vi "Autonomous Independent.vi"   [LabVIEW 2017]
doc: "This VI is called when autonomous begins, and will automatically be terminated when autonomous ends. You can carry out timed or sensor driven robot movement independently without needing to return to the caller."
uses:
  <vilib>/Rock Robotics/WPI/Utilities/WPI_GetSetVariantRefNum.vi
  Robot Global Data.vi
panel:
  # "Be sure to right-click and choose Data Operations>>Make Current Value default if you want to save the array values with the VI"
types:
  T1 = enum16{"Manual", "Turn For Angle", "Drive For Distance", "Motion Profile", "Recorded Auto File"}
  T2 = enum16{"Manual", "Turn For Angle", "Drive For Distance", "Motion Profile"}
  T3 = typedef "WPI_JoystickDevRef.ctl" = cluster{"Device":T4}
  T4 = typedef "WPI_JoystickDeviceEnum.ctl" = enum16{"USB 0", "USB 1", "USB 2", "USB 3", "USB 4", "USB 5"}
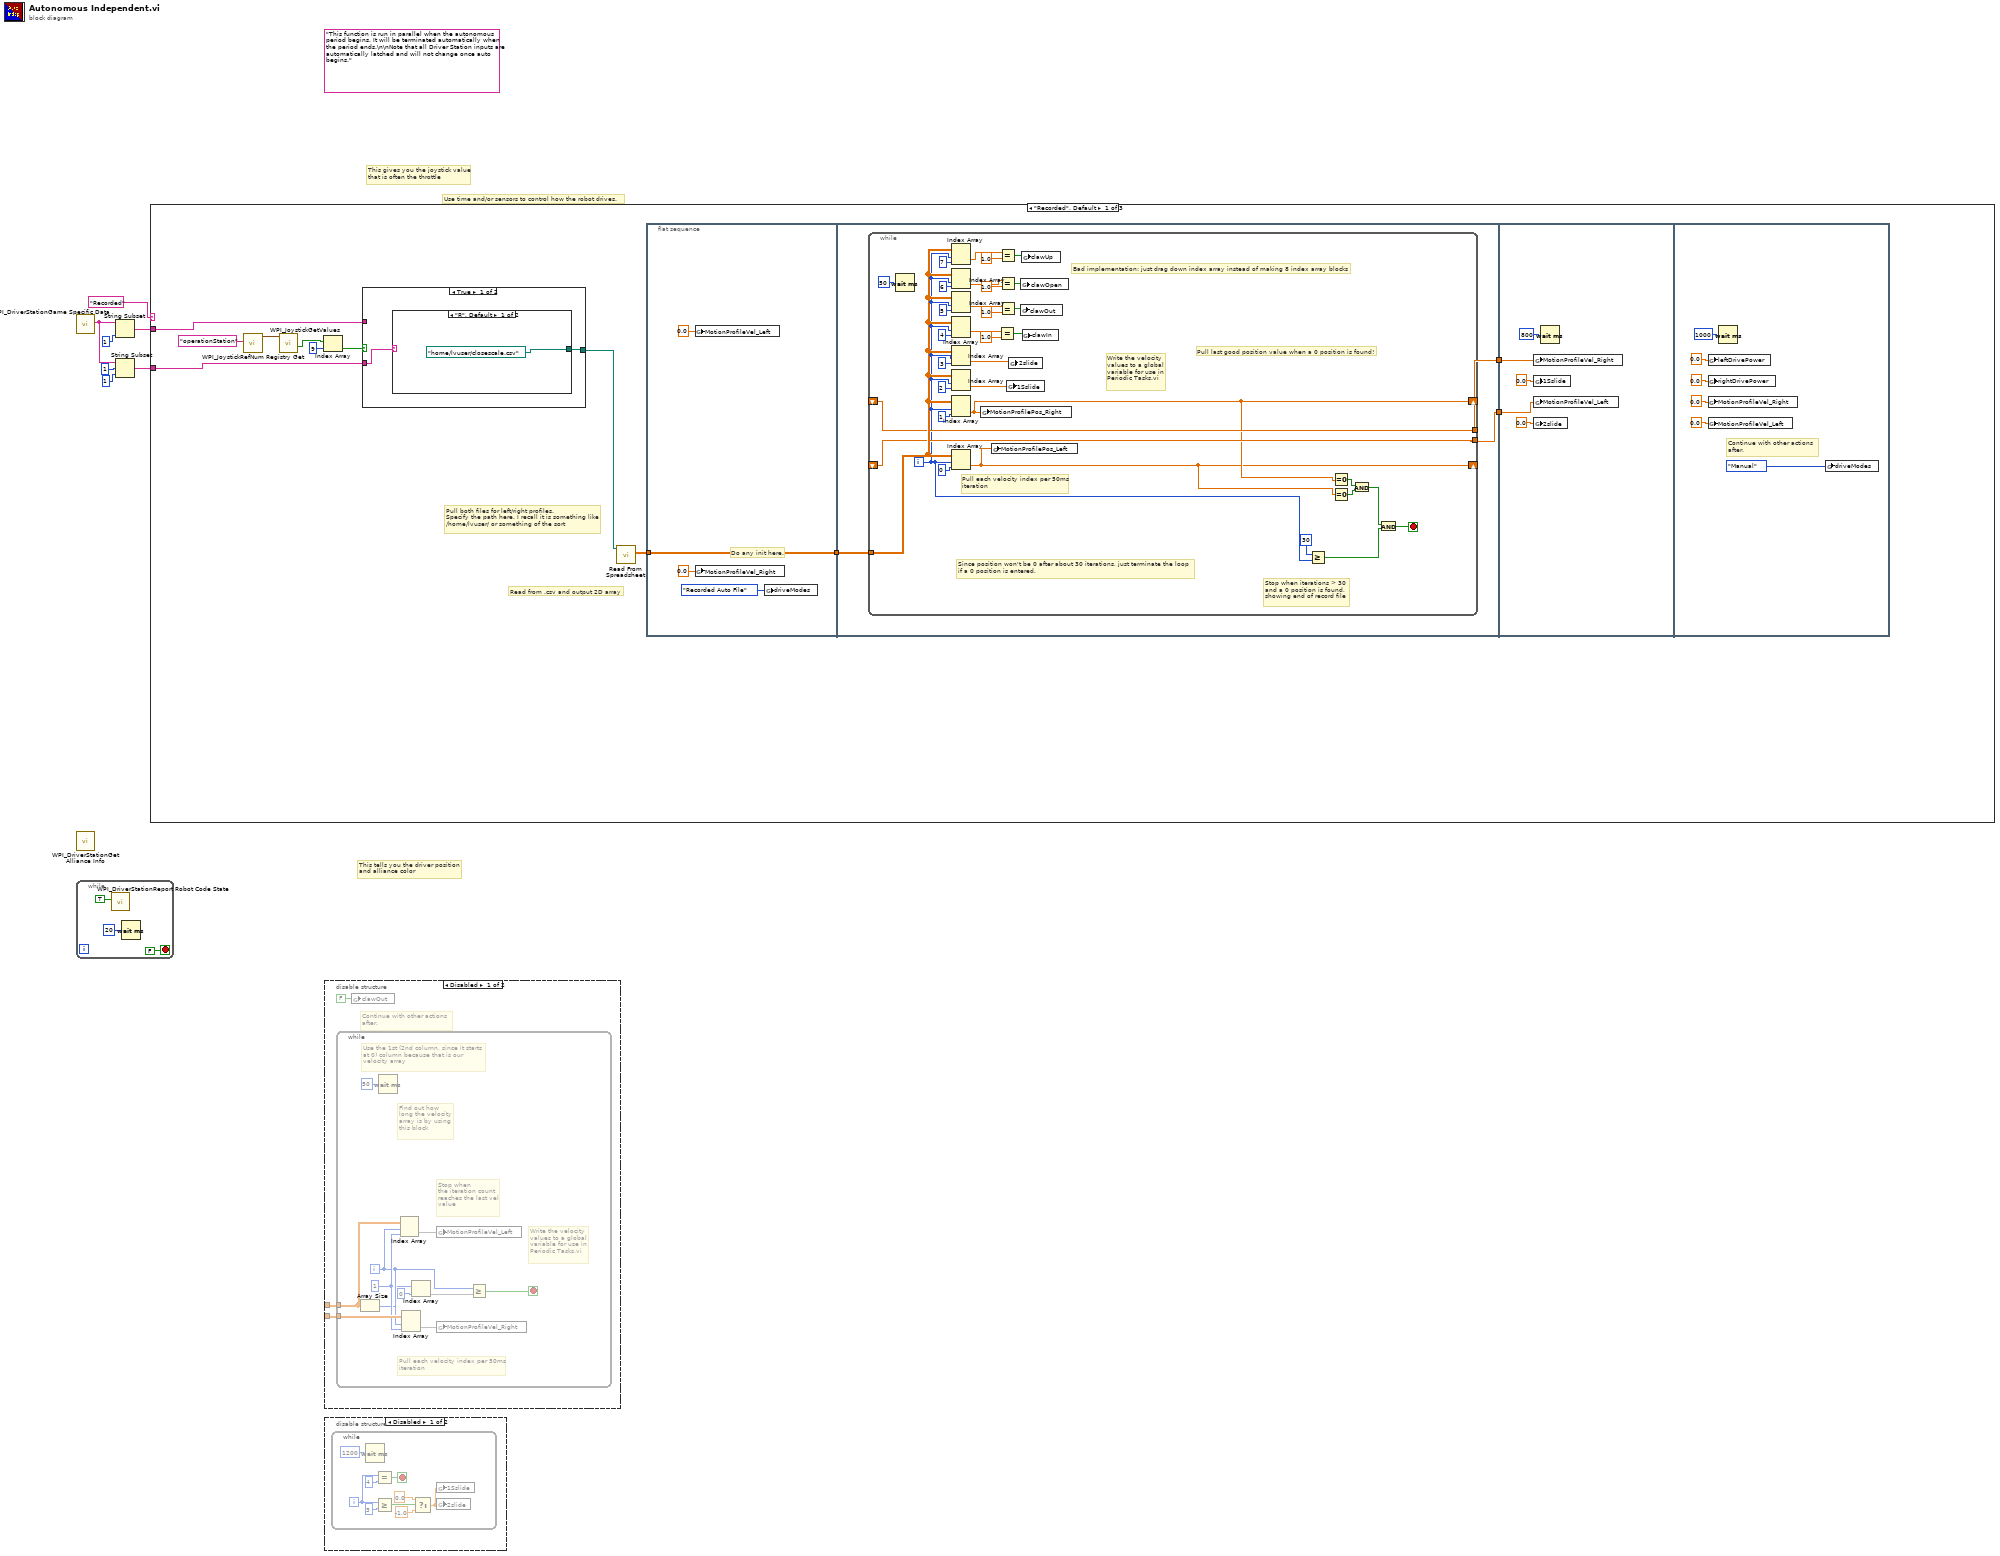
[diagram p0: block diagram]
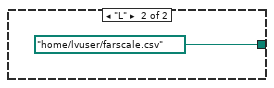
[diagram p2: hidden frame]
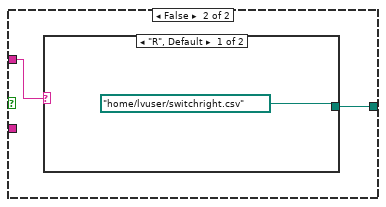
[diagram p3: hidden frame]
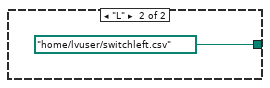
[diagram p4: hidden frame]
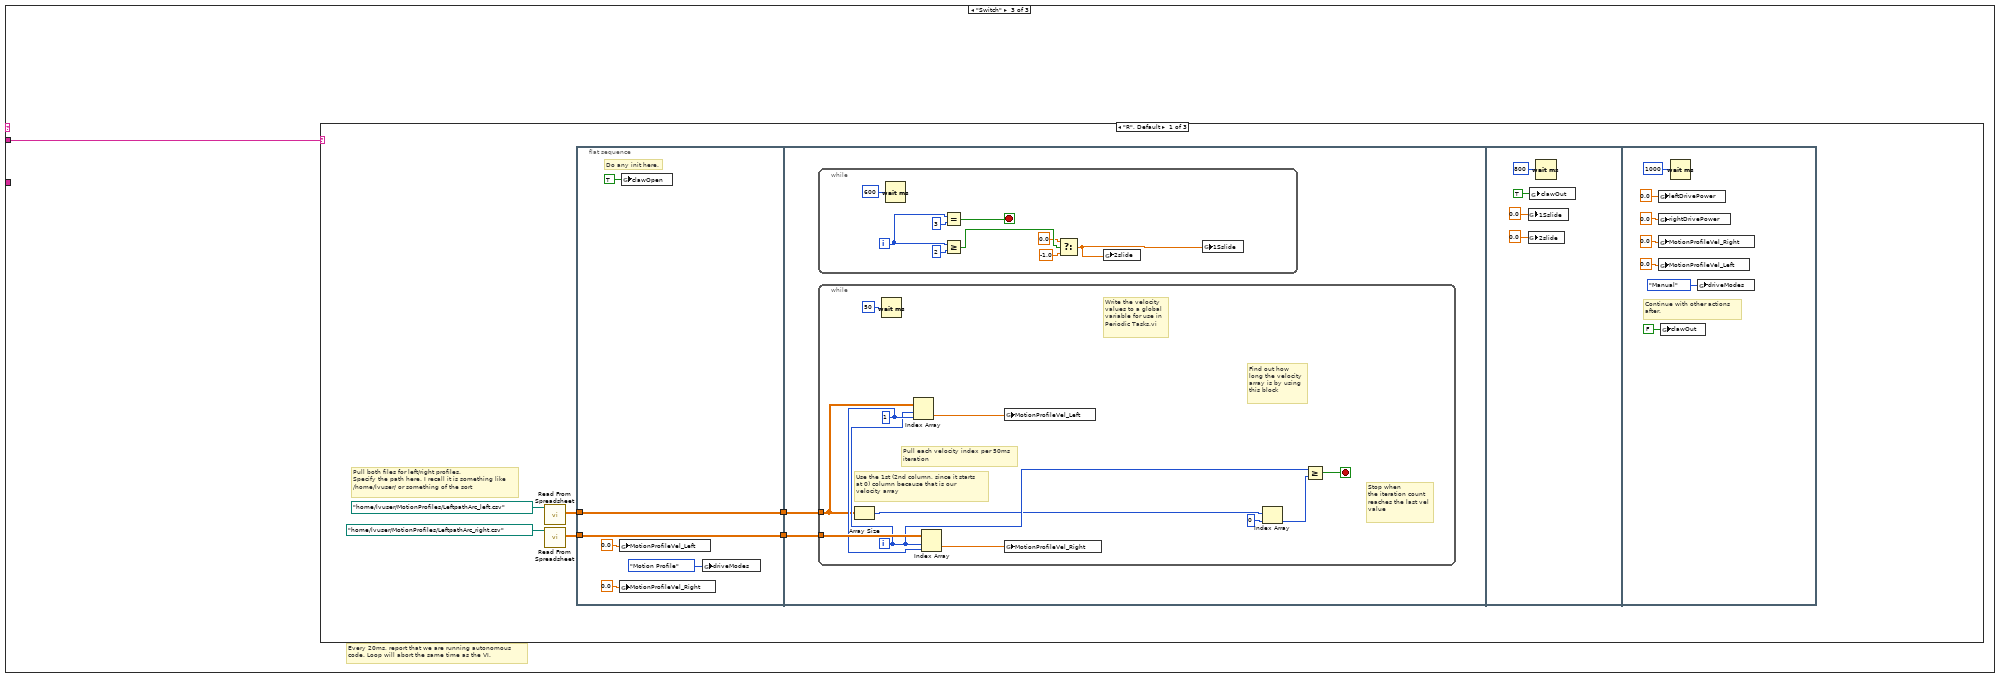
[diagram p6: hidden frame]
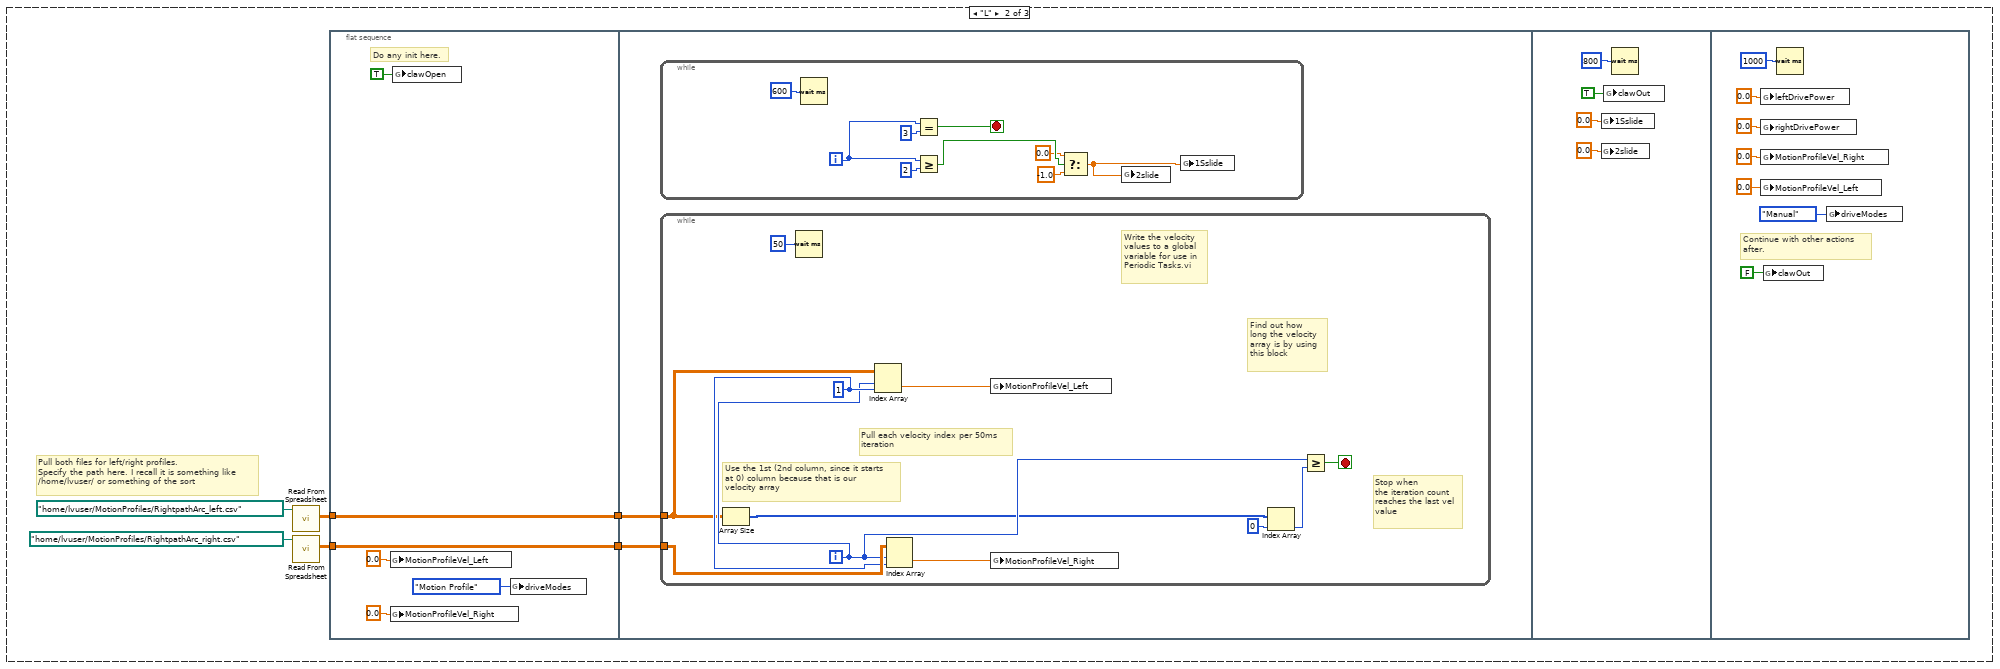
[diagram p7: hidden frame]
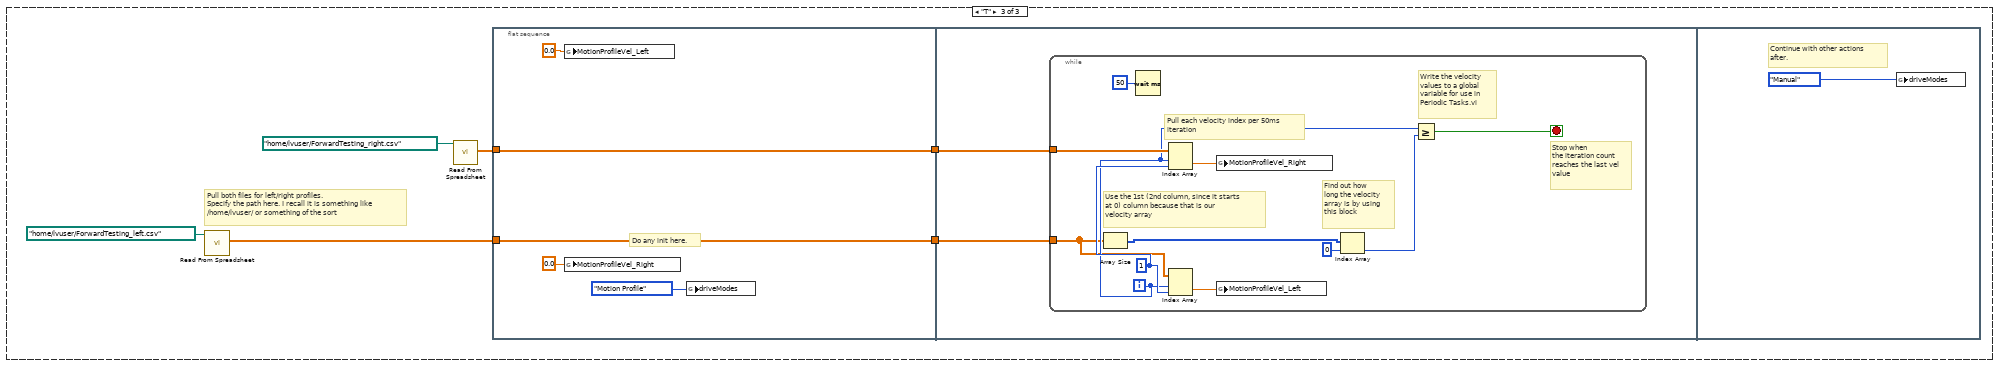
[diagram p8: hidden frame]
diagram:
  (unwired) "This function is run in parallel when the autonomous period begins. It will be terminated automatically when the period ends.\n\nNote that all Driver Station inputs are automatically latched and will not change once auto begins."
  # "This gives you the joystick value\nthat is often the throttle"
  # "Use time and/or sensors to control how the robot drives."
  # "This tells you the driver position\nand alliance color"
  n1 = call <vilib>:"WPI_DriverStationGame Specific Data.vi"() -> ("Game Specific Data"=w4:string)  [unwired: 11 in]
  n2 = call <vilib>:"WPI_DriverStationGet Alliance Info.vi"() -> ()  [unwired: 12 out]
  n3 = while {
    stop <- FALSE stop-if-true
    n4 = call <vilib>:"WPI_DriverStationReport Robot Code State.vi"("Autonomous"=TRUE) -> ()  [unwired: 10 in, 1 out]
    n5 = Wait (ms)(milliseconds to wait=u32 20) -> ()  [unwired: 1 out]
  }
  n6 = String Subset(string=w4, length (rest)=1 ("length (rest)")) -> (substring=w7:string)  [unwired: 1 in]
  n7 = String Subset(string=w4, offset (0)=1, length (rest)=1 ("length (rest)")) -> (substring=w3:string)
  n8 = case shown="\"Recorded\", Default" "Recorded" {
    tunnel: w7 -> [w20 _ w84]
    tunnel: w3 -> [w19 _ _]
    frame "Recorded", Default {
      # "Read from .csv and output 2D array"
      # "Pull both files for left/right profiles.\nSpecify the path here. I recall it is something like\n/home/lvuser/ or something of the sort"
      n9 = call <vilib>:"WPI_JoystickRefNum Registry Get.vi"("refnum name"="operationStation") -> ("JoystickDevRef"=w16:T3)  [unwired: 1 in, 9 out]
      n10 = call <vilib>:"WPI_JoystickGetValues.vi"("JoystickDevRef"=w16) -> ("Buttons"=w17:bool[])  [unwired: 6 in, 4 out]
      n11 = Index Array(array=w17, index=9) -> (element=w13:bool)
      n12 = case shown="True" w13 {
        tunnel: w20 -> [_ w28]
        tunnel: w19 -> [w24 _]
        tunnel: [w23 w27] -> w18
        frame True {
          n13 = case shown="\"R\", Default" w24 {
            tunnel: [path "/home/lvuser/closescale.csv" ("Spreadsheet path (.csv)") path "/home/lvuser/farscale.csv" ("Spreadsheet path (.csv)")] -> w23
            frame "R", Default {
            }
            frame "L" {
            }
          }
        }
        frame False {
          n14 = case shown="\"R\", Default" w28 {
            tunnel: [path "/home/lvuser/switchright.csv" ("Spreadsheet path (.csv)") path "/home/lvuser/switchleft.csv" ("Spreadsheet path (.csv)")] -> w27
            frame "R", Default {
            }
            frame "L" {
            }
          }
        }
      }
      n15 = call "Read From Spreadsheet.vi"("Spreadsheet path (.csv)"=w18) -> ("Data Dsiplay"=w21:dbl[][])  [unwired: 9 in, 1 out]
      n16 = flat-sequence {
        tunnel: w21 -> [w34]
        tunnel: [w34] -> w22
        tunnel: w22 -> [w37]
        tunnel: [w36] -> w12
        tunnel: [w35] -> w11
        tunnel: w12 -> [w74]
        tunnel: w11 -> [w73]
        frame #0 {
          # "Do any init here."
          n17 = global write "Robot Global Data.vi" "MotionProfileVel_Left"(0.0 ("MotionProfileVel_Left")) -> ()
          n18 = global write "Robot Global Data.vi" "MotionProfileVel_Right"(0.0 ("MotionProfileVel_Right")) -> ()
          n19 = global write "Robot Global Data.vi" "driveModes"(T1."Recorded Auto File" ("driveModes")) -> ()
        }
        frame #1 {
          n20 = while {
            tunnel: w37 -> [w63]
            shift-right: [w43] -> _
            shift-left: _ -> [w47]
            shift-right: [w44] -> _
            shift-left: _ -> [w48]
            tunnel: [w48] -> w36
            tunnel: [w47] -> w35
            i -> [w46]
            stop <- w38 stop-if-true
            # "Pull last good position value when a 0 position is found!"
            # "Since position won't be 0 after about 30 iterations, just terminate the loop \nif a 0 position is entered."
            # "Bad implementation: just drag down index array instead of making 8 index array blocks"
            # "Write the velocity \nvalues to a global\nvariable for use in\nPeriodic Tasks.vi"
            # "Stop when iterations > 30\nand a 0 position is found, \nshowing end of record file"
            # "Pull each velocity index per 50ms\niteration"
            n21 = Wait (ms)(milliseconds to wait=u32 50) -> ()  [unwired: 1 out]
            n22 = Index Array(array=w63, index (row)=w46, index (col)=4 ("disabled index (col)")) -> (element=w60:dbl)
            n23 = Index Array(array=w63, index (row)=w46, index (col)=3 ("disabled index (col)")) -> (element=w61:dbl)
            n24 = Index Array(array=w63, index (row)=w46, index (col)=2 ("index (row)")) -> (element=w62:dbl)
            n25 = Index Array(array=w63, index (row)=w46, index (col)=7 ("disabled index (col)")) -> (element=w57:dbl)
            n26 = Index Array(array=w63, index (row)=w46, index (col)=6 ("disabled index (col)")) -> (element=w58:dbl)
            n27 = Index Array(array=w63, index (row)=w46, index (col)=5 ("disabled index (col)")) -> (element=w59:dbl)
            n28 = Index Array(array=w63, index (row)=w46, index (col)=1) -> (element=w44:dbl)
            n29 = Index Array(array=w63, index (row)=w46, index (col)=0 ("disabled index (col)")) -> (element=w43:dbl)
            n30 = global write "Robot Global Data.vi" "MotionProfilePos_Right"(w44) -> ()
            n31 = global write "Robot Global Data.vi" "MotionProfilePos_Left"(w43) -> ()
            n32 = Equal?(x=w60, y=1.0) -> (x = y?=w49:bool)
            n33 = Equal?(x=w57, y=1.0) -> (x = y?=w52:bool)
            n34 = Equal?(x=w58, y=1.0) -> (x = y?=w51:bool)
            n35 = Equal?(x=w59, y=1.0) -> (x = y?=w50:bool)
            n36 = global write "Robot Global Data.vi" "1Sslide"(w62) -> ()
            n37 = global write "Robot Global Data.vi" "2slide"(w61) -> ()
            n38 = global write "Robot Global Data.vi" "clawOut"(w50) -> ()
            n39 = global write "Robot Global Data.vi" "clawOpen"(w51) -> ()
            n40 = global write "Robot Global Data.vi" "clawUp"(w52) -> ()
            n41 = global write "Robot Global Data.vi" "clawIn"(w49) -> ()
            n42 = Greater Or Equal?(x=30, y=w46) -> (x >= y?=w40:bool)
            n43 = Equal To 0?(x=w44) -> (x = 0?=w41:bool)
            n44 = Equal To 0?(x=w43) -> (x = 0?=w42:bool)
            n45 = And(x=w41, y=w42) -> (x .and. y?=w39:bool)
            n46 = And(x=w39, y=w40) -> (x .and. y?=w38:bool)
          }
        }
        frame #2 {
          n47 = global write "Robot Global Data.vi" "MotionProfileVel_Right"(w74) -> ()
          n48 = global write "Robot Global Data.vi" "1Sslide"(0.0 ("1Sslide")) -> ()
          n49 = global write "Robot Global Data.vi" "MotionProfileVel_Left"(w73) -> ()
          n50 = global write "Robot Global Data.vi" "2slide"(0.0 ("2slide")) -> ()
          n51 = Wait (ms)(milliseconds to wait=u32 800) -> ()  [unwired: 1 out]
        }
        frame #3 {
          # "Continue with other actions\nafter."
          n52 = global write "Robot Global Data.vi" "leftDrivePower"(0.0 ("MotionProfileVel_Right")) -> ()
          n53 = global write "Robot Global Data.vi" "rightDrivePower"(0.0 ("MotionProfileVel_Left")) -> ()
          n54 = global write "Robot Global Data.vi" "MotionProfileVel_Right"(0.0 ("MotionProfileVel_Right")) -> ()
          n55 = global write "Robot Global Data.vi" "MotionProfileVel_Left"(0.0 ("MotionProfileVel_Left")) -> ()
          n56 = Wait (ms)(milliseconds to wait=u32 1000) -> ()  [unwired: 1 out]
          n57 = global write "Robot Global Data.vi" "driveModes"(T2."Manual" ("driveModes")) -> ()
        }
      }
    }
    frame "Straight" {
    }
    frame "Switch" {
      # "Every 20ms, report that we are running autonomous\ncode. Loop will abort the same time as the VI."
      n58 = case shown="\"R\", Default" w84 {
        frame "R", Default {
          # "Pull both files for left/right profiles.\nSpecify the path here. I recall it is something like\n/home/lvuser/ or something of the sort"
          n59 = call "Read From Spreadsheet.vi"("Spreadsheet path (.csv)"=path "/home/lvuser/MotionProfiles/LeftpathArc_left.csv") -> ("Data Dsiplay"=w86:dbl[][])  [unwired: 9 in, 1 out]
          n60 = call "Read From Spreadsheet.vi"("Spreadsheet path (.csv)"=path "/home/lvuser/MotionProfiles/LeftpathArc_right.csv") -> ("Data Dsiplay"=w85:dbl[][])  [unwired: 9 in, 1 out]
          n61 = flat-sequence {
            tunnel: w85 -> [w95]
            tunnel: w86 -> [w96]
            tunnel: [w96] -> w88
            tunnel: [w95] -> w87
            tunnel: w88 -> [w98]
            tunnel: w87 -> [w97]
            frame #0 {
              # "Do any init here."
              n62 = global write "Robot Global Data.vi" "MotionProfileVel_Left"(0.0 ("MotionProfileVel_Left")) -> ()
              n63 = global write "Robot Global Data.vi" "MotionProfileVel_Right"(0.0 ("MotionProfileVel_Right")) -> ()
              n64 = global write "Robot Global Data.vi" "clawOpen"(TRUE ("clawOpen")) -> ()
              n65 = global write "Robot Global Data.vi" "driveModes"(T2."Motion Profile" ("driveModes")) -> ()
            }
            frame #1 {
              n66 = while {
                i -> [w100]
                stop <- w102 stop-if-true
                n67 = Wait (ms)(milliseconds to wait=u32 600) -> ()  [unwired: 1 out]
                n68 = Equal?(x=w100, y=3) -> (x = y?=w102:bool)
                n69 = Greater Or Equal?(x=w100, y=2) -> (x >= y?=w106:bool)
                n70 = Select(t=0.0, s=w106, f=-1.0) -> (s? t:f=w103:dbl)
                n71 = global write "Robot Global Data.vi" "2slide"(w103) -> ()
                n72 = global write "Robot Global Data.vi" "1Sslide"(w103) -> ()
              }
              n73 = while {
                tunnel: w98 -> [w113]
                tunnel: w97 -> [w118]
                i -> [w114]
                stop <- w109 stop-if-true
                w117 = 1 ("disabled index (col)")
                # "Write the velocity \nvalues to a global\nvariable for use in\nPeriodic Tasks.vi"
                # "Find out how\nlong the velocity\narray is by using \nthis block"
                # "Stop when \nthe iteration count\nreaches the last vel\nvalue"
                # "Use the 1st (2nd column, since it starts\nat 0) column because that is our\nvelocity array"
                # "Pull each velocity index per 50ms\niteration"
                n74 = Array Size(array=w113) -> (size(s)=w112:i32[])
                n75 = Wait (ms)(milliseconds to wait=u32 50) -> ()  [unwired: 1 out]
                n76 = Index Array(array=w113, index (row)=w114, index (col)=w117) -> (element=w115:dbl)
                n77 = Index Array(array=w118, index (row)=w114, index (col)=w117) -> (element=w116:dbl)
                n78 = global write "Robot Global Data.vi" "MotionProfileVel_Left"(w115) -> ()
                n79 = global write "Robot Global Data.vi" "MotionProfileVel_Right"(w116) -> ()
                n80 = Index Array(array=w112, index=0) -> (element=w110:i32)
                n81 = Greater Or Equal?(x=w114, y=w110) -> (x >= y?=w109:bool)
              }
            }
            frame #2 {
              n82 = global write "Robot Global Data.vi" "1Sslide"(0.0 ("1Sslide")) -> ()
              n83 = global write "Robot Global Data.vi" "2slide"(0.0 ("2slide")) -> ()
              n84 = global write "Robot Global Data.vi" "clawOut"(TRUE ("clawOut")) -> ()
              n85 = Wait (ms)(milliseconds to wait=u32 800) -> ()  [unwired: 1 out]
            }
            frame #3 {
              # "Continue with other actions\nafter."
              n86 = global write "Robot Global Data.vi" "leftDrivePower"(0.0 ("MotionProfileVel_Right")) -> ()
              n87 = global write "Robot Global Data.vi" "rightDrivePower"(0.0 ("MotionProfileVel_Left")) -> ()
              n88 = global write "Robot Global Data.vi" "MotionProfileVel_Right"(0.0 ("MotionProfileVel_Right")) -> ()
              n89 = global write "Robot Global Data.vi" "MotionProfileVel_Left"(0.0 ("MotionProfileVel_Left")) -> ()
              n90 = global write "Robot Global Data.vi" "clawOut"(FALSE ("clawOut")) -> ()
              n91 = Wait (ms)(milliseconds to wait=u32 1000) -> ()  [unwired: 1 out]
              n92 = global write "Robot Global Data.vi" "driveModes"(T2."Manual" ("driveModes")) -> ()
            }
          }
        }
        frame "L" {
          # "Pull both files for left/right profiles.\nSpecify the path here. I recall it is something like\n/home/lvuser/ or something of the sort"
          n93 = call "Read From Spreadsheet.vi"("Spreadsheet path (.csv)"=path "/home/lvuser/MotionProfiles/RightpathArc_left.csv") -> ("Data Dsiplay"=w131:dbl[][])  [unwired: 9 in, 1 out]
          n94 = call "Read From Spreadsheet.vi"("Spreadsheet path (.csv)"=path "/home/lvuser/MotionProfiles/RightpathArc_right.csv") -> ("Data Dsiplay"=w130:dbl[][])  [unwired: 9 in, 1 out]
          n95 = flat-sequence {
            tunnel: w130 -> [w140]
            tunnel: w131 -> [w141]
            tunnel: [w141] -> w135
            tunnel: [w140] -> w134
            tunnel: w135 -> [w143]
            tunnel: w134 -> [w142]
            frame #0 {
              # "Do any init here."
              n96 = global write "Robot Global Data.vi" "MotionProfileVel_Left"(0.0 ("MotionProfileVel_Left")) -> ()
              n97 = global write "Robot Global Data.vi" "MotionProfileVel_Right"(0.0 ("MotionProfileVel_Right")) -> ()
              n98 = global write "Robot Global Data.vi" "clawOpen"(TRUE ("clawOpen")) -> ()
              n99 = global write "Robot Global Data.vi" "driveModes"(T2."Motion Profile" ("driveModes")) -> ()
            }
            frame #1 {
              n100 = while {
                i -> [w145]
                stop <- w147 stop-if-true
                n101 = Wait (ms)(milliseconds to wait=u32 600) -> ()  [unwired: 1 out]
                n102 = Equal?(x=w145, y=3) -> (x = y?=w147:bool)
                n103 = Greater Or Equal?(x=w145, y=2) -> (x >= y?=w151:bool)
                n104 = Select(t=0.0, s=w151, f=-1.0) -> (s? t:f=w148:dbl)
                n105 = global write "Robot Global Data.vi" "2slide"(w148) -> ()
                n106 = global write "Robot Global Data.vi" "1Sslide"(w148) -> ()
              }
              n107 = while {
                tunnel: w143 -> [w158]
                tunnel: w142 -> [w163]
                i -> [w159]
                stop <- w154 stop-if-true
                w162 = 1 ("disabled index (col)")
                # "Write the velocity \nvalues to a global\nvariable for use in\nPeriodic Tasks.vi"
                # "Find out how\nlong the velocity\narray is by using \nthis block"
                # "Stop when \nthe iteration count\nreaches the last vel\nvalue"
                # "Use the 1st (2nd column, since it starts\nat 0) column because that is our\nvelocity array"
                # "Pull each velocity index per 50ms\niteration"
                n108 = Array Size(array=w158) -> (size(s)=w157:i32[])
                n109 = Wait (ms)(milliseconds to wait=u32 50) -> ()  [unwired: 1 out]
                n110 = Index Array(array=w158, index (row)=w159, index (col)=w162) -> (element=w160:dbl)
                n111 = Index Array(array=w163, index (row)=w159, index (col)=w162) -> (element=w161:dbl)
                n112 = global write "Robot Global Data.vi" "MotionProfileVel_Left"(w160) -> ()
                n113 = global write "Robot Global Data.vi" "MotionProfileVel_Right"(w161) -> ()
                n114 = Index Array(array=w157, index=0) -> (element=w155:i32)
                n115 = Greater Or Equal?(x=w159, y=w155) -> (x >= y?=w154:bool)
              }
            }
            frame #2 {
              n116 = global write "Robot Global Data.vi" "1Sslide"(0.0 ("1Sslide")) -> ()
              n117 = global write "Robot Global Data.vi" "2slide"(0.0 ("2slide")) -> ()
              n118 = global write "Robot Global Data.vi" "clawOut"(TRUE ("clawOut")) -> ()
              n119 = Wait (ms)(milliseconds to wait=u32 800) -> ()  [unwired: 1 out]
            }
            frame #3 {
              # "Continue with other actions\nafter."
              n120 = global write "Robot Global Data.vi" "leftDrivePower"(0.0 ("MotionProfileVel_Right")) -> ()
              n121 = global write "Robot Global Data.vi" "rightDrivePower"(0.0 ("MotionProfileVel_Left")) -> ()
              n122 = global write "Robot Global Data.vi" "MotionProfileVel_Right"(0.0 ("MotionProfileVel_Right")) -> ()
              n123 = global write "Robot Global Data.vi" "MotionProfileVel_Left"(0.0 ("MotionProfileVel_Left")) -> ()
              n124 = global write "Robot Global Data.vi" "clawOut"(FALSE ("clawOut")) -> ()
              n125 = Wait (ms)(milliseconds to wait=u32 1000) -> ()  [unwired: 1 out]
              n126 = global write "Robot Global Data.vi" "driveModes"(T2."Manual" ("driveModes")) -> ()
            }
          }
        }
        frame "T" {
          # "Pull both files for left/right profiles.\nSpecify the path here. I recall it is something like\n/home/lvuser/ or something of the sort"
          n127 = call "Read From Spreadsheet.vi"("Spreadsheet path (.csv)"=path "/home/lvuser/ForwardTesting_left.csv") -> ("Data Dsiplay"=w178:dbl[][])  [unwired: 9 in, 1 out]
          n128 = call "Read From Spreadsheet.vi"("Spreadsheet path (.csv)"=path "/home/lvuser/ForwardTesting_right.csv") -> ("Data Dsiplay"=w177:dbl[][])  [unwired: 9 in, 1 out]
          n129 = flat-sequence {
            tunnel: w177 -> [w184]
            tunnel: w178 -> [w185]
            tunnel: [w185] -> w176
            tunnel: [w184] -> w175
            tunnel: w176 -> [w187]
            tunnel: w175 -> [w186]
            frame #0 {
              # "Do any init here."
              n130 = global write "Robot Global Data.vi" "MotionProfileVel_Left"(0.0 ("MotionProfileVel_Left")) -> ()
              n131 = global write "Robot Global Data.vi" "MotionProfileVel_Right"(0.0 ("MotionProfileVel_Right")) -> ()
              n132 = global write "Robot Global Data.vi" "driveModes"(T2."Motion Profile" ("driveModes")) -> ()
            }
            frame #1 {
              n133 = while {
                tunnel: w187 -> [w193]
                tunnel: w186 -> [w198]
                i -> [w194]
                stop <- w189 stop-if-true
                w197 = 1 ("disabled index (col)")
                # "Write the velocity \nvalues to a global\nvariable for use in\nPeriodic Tasks.vi"
                # "Find out how\nlong the velocity\narray is by using \nthis block"
                # "Stop when \nthe iteration count\nreaches the last vel\nvalue"
                # "Use the 1st (2nd column, since it starts\nat 0) column because that is our\nvelocity array"
                # "Pull each velocity index per 50ms\niteration"
                n134 = Array Size(array=w193) -> (size(s)=w192:i32[])
                n135 = Wait (ms)(milliseconds to wait=u32 50) -> ()  [unwired: 1 out]
                n136 = Index Array(array=w198, index (row)=w194, index (col)=w197) -> (element=w196:dbl)
                n137 = Index Array(array=w193, index (row)=w194, index (col)=w197) -> (element=w195:dbl)
                n138 = global write "Robot Global Data.vi" "MotionProfileVel_Right"(w196) -> ()
                n139 = global write "Robot Global Data.vi" "MotionProfileVel_Left"(w195) -> ()
                n140 = Index Array(array=w192, index=0) -> (element=w190:i32)
                n141 = Greater Or Equal?(x=w194, y=w190) -> (x >= y?=w189:bool)
              }
            }
            frame #2 {
              # "Continue with other actions\nafter."
              n142 = global write "Robot Global Data.vi" "driveModes"(T2."Manual" ("driveModes")) -> ()
            }
          }
        }
      }
    }
  }
  n143 = disable-structure shown="Disabled" {
    disable-tunnel: _ -> [w201 _]
    disable-tunnel: _ -> [w200 _]
    frame Disabled {
      # "Continue with other actions\nafter."
      n144 = while {
        tunnel: w201 -> [w207]
        tunnel: w200 -> [w212]
        i -> [w208]
        stop <- w203 stop-if-true
        w211 = 1 ("disabled index (col)")
        # "Write the velocity \nvalues to a global\nvariable for use in\nPeriodic Tasks.vi"
        # "Find out how\nlong the velocity\narray is by using \nthis block"
        # "Stop when \nthe iteration count\nreaches the last vel\nvalue"
        # "Use the 1st (2nd column, since it starts\nat 0) column because that is our\nvelocity array"
        # "Pull each velocity index per 50ms\niteration"
        n145 = Array Size(array=w207) -> (size(s)=w206:i32)
        n146 = Wait (ms)(milliseconds to wait=u32 50) -> ()  [unwired: 1 out]
        n147 = Index Array(array=w207, index (row)=w208, index (col)=w211) -> (element=w209)
        n148 = Index Array(array=w212, index (row)=w208, index (col)=w211) -> (element=w210)
        n149 = Index Array(array=w206, index=0) -> (element=w204)
        n150 = global write "Robot Global Data.vi" "MotionProfileVel_Left"(w209) -> ()
        n151 = global write "Robot Global Data.vi" "MotionProfileVel_Right"(w210) -> ()
        n152 = Greater Or Equal?(x=w208, y=w204) -> (x >= y?=w203:bool)
      }
      n153 = global write "Robot Global Data.vi" "clawOut"(FALSE ("clawOpen")) -> ()
    }
    frame Enabled {
    }
  }
  n154 = disable-structure shown="Disabled" {
    frame Disabled {
      n155 = while {
        i -> [w215]
        stop <- w217 stop-if-true
        n156 = Wait (ms)(milliseconds to wait=u32 1200) -> ()  [unwired: 1 out]
        n157 = Equal?(x=w215, y=4) -> (x = y?=w217:bool)
        n158 = Greater Or Equal?(x=w215, y=3) -> (x >= y?=w221:bool)
        n159 = Select(t=0.0, s=w221, f=-1.0) -> (s? t:f=w218:dbl)
        n160 = global write "Robot Global Data.vi" "1Sslide"(w218) -> ()
        n161 = global write "Robot Global Data.vi" "2slide"(w218) -> ()
      }
    }
    frame Enabled {
    }
  }
